vi "Set Custom Window Size.vi"(8 "error in (no error)":errorcluster, 9 "Custom Window Size":cluster{"Height":i16, "Width":i16}={"Height"=-1, "Width"=-1}, 10 "Custom Window Position":cluster{"Top":i16, "Left":i16}={"Top"=-1, "Left"=-1}, 11 "VI in":refnum<vi>) -> (0 "error out":errorcluster, 3 "VI out":refnum<vi>)   [LabVIEW 2017, in "IViewable.lvlib" / "IViewable.lvclass"]
uses:
  IViewable.lvclass
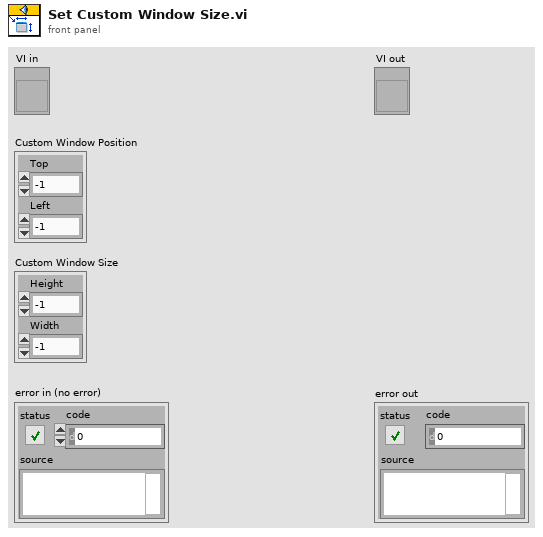
[diagram p1: front panel]
types:
  T1 = typedef "LVRectTypeDef.ctl" = cluster{"Left":i16, "Top":i16, "Right":i16, "Bottom":i16}
  T2 = typedef "LVPointTypeDef.ctl" = cluster{"Horizontal":i16, "Vertical":i16}
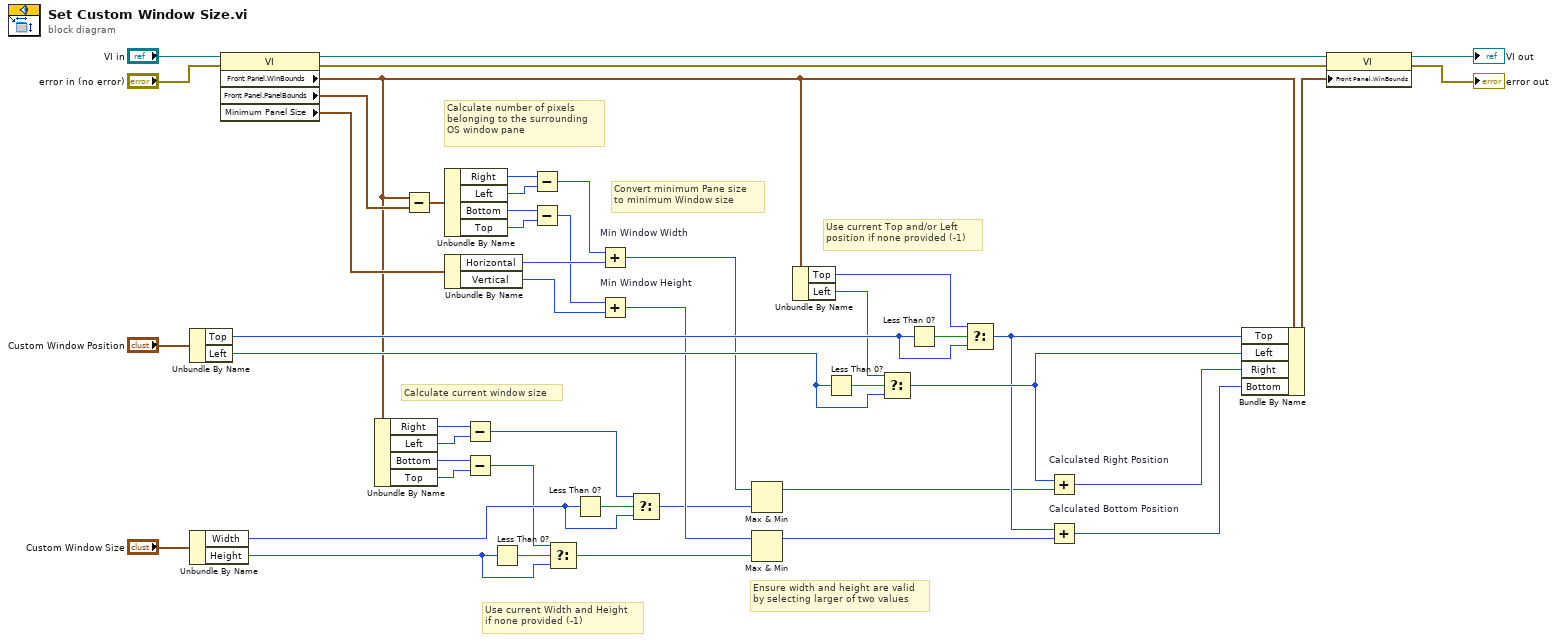
[diagram p0: block diagram]
diagram:
  # "Use current Width and Height\nif none provided (-1)"
  # "Calculate current window size"
  # "Ensure width and height are valid\nby selecting larger of two values"
  # "Convert minimum Pane size\nto minimum Window size"
  # "Calculate number of pixels\nbelonging to the surrounding\nOS window pane"
  # "Use current Top and/or Left\nposition if none provided (-1)"
  n1 = Unbundle By Name("Custom Window Position") -> ("Top"=w36:i16, "Left"=w34:i16)
  n2 = Unbundle By Name("Custom Window Size") -> ("Width"=w10:i16, "Height"=w11:i16)
  n3 = property class="VI"(reference="VI in", error in="error in (no error)") -> (reference out=w39:refnum<vi>, error out=w41:errorcluster, "Front Panel.WinBounds"=w7:T1, "Front Panel.PanelBounds"=w32:T1, "Minimum Panel Size"=w26:T2)
  n4 = Unbundle By Name(w7) -> ("Right"=w6:i16, "Left"=w4:i16, "Bottom"=w5:i16, "Top"=w3:i16)
  n5 = Subtract(x=w7, y=w32) -> (x-y=w31:T1)
  n6 = Unbundle By Name(w31) -> ("Right"=w30:i16, "Left"=w29:i16, "Bottom"=w28:i16, "Top"=w27:i16)
  n7 = Unbundle By Name(w26) -> ("Horizontal"=w25:i16, "Vertical"=w24:i16)
  n8 = Subtract(x=w6, y=w4) -> (x-y=w2:i16)
  n9 = Subtract(x=w5, y=w3) -> (x-y=w1:i16)
  n10 = Less Than 0?(x=w11) -> (x < 0?=w13:bool)
  n11 = Subtract(x=w30, y=w29) -> (x-y=w23:i16)
  n12 = Subtract(x=w28, y=w27) -> (x-y=w22:i16)
  n13 = Select(t=w1, s=w13, f=w11) -> (s? t:f=w8:i16)
  n14 = Less Than 0?(x=w10) -> (x < 0?=w12:bool)
  n15 = Add "Min Window Width"(x=w23, y=w25) -> (x+y=w15:i16)
  n16 = Add "Min Window Height"(x=w22, y=w24) -> (x+y=w17:i16)
  n17 = Select(t=w2, s=w12, f=w10) -> (s? t:f=w9:i16)
  n18 = Max & Min(x=w15, y=w9) -> (max(x,y)=w14:i16)  [unwired: 1 out]
  n19 = Max & Min(x=w17, y=w8) -> (max(x,y)=w16:i16)  [unwired: 1 out]
  n20 = Unbundle By Name(w7) -> ("Top"=w37:i16, "Left"=w33:i16)
  n21 = Less Than 0?(x=w34) -> (x < 0?=w35:bool)
  n22 = Select(t=w33, s=w35, f=w34) -> (s? t:f=w21:i16)
  n23 = Less Than 0?(x=w36) -> (x < 0?=w38:bool)
  n24 = Select(t=w37, s=w38, f=w36) -> (s? t:f=w20:i16)
  n25 = Add "Calculated Right Position"(x=w21, y=w14) -> (x+y=w19:i16)
  n26 = Add "Calculated Bottom Position"(x=w20, y=w16) -> (x+y=w18:i16)
  n27 = Bundle By Name(cluster=w7, "Top"=w20, "Left"=w21, "Right"=w19, "Bottom"=w18) -> (w47:T1)
  n28 = property class="VI"(reference=w39, error in=w41, "Front Panel.WinBounds"=w47) -> (reference out=→"VI out":refnum<vi>, error out=→"error out":errorcluster)
